vi "Lectura de datos 2.vi"() -> ()   [LabVIEW 2020]
panel:
  out "Graficacion señales":dynamicdata(graph)
  in  "stop":bool
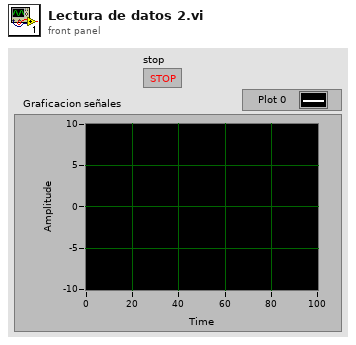
[diagram p1: front panel]
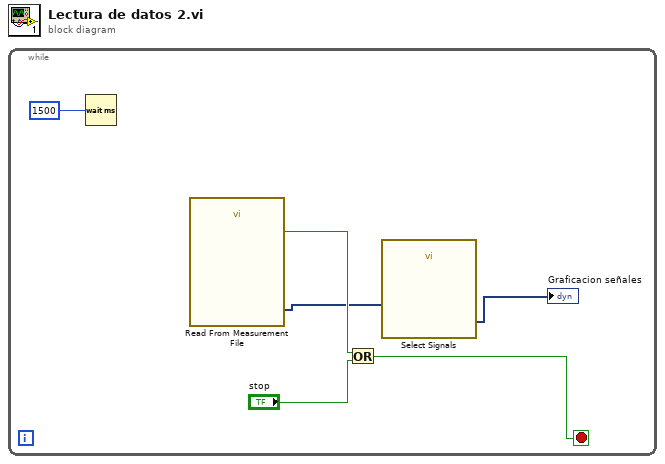
[diagram p0: block diagram]
diagram:
  n1 = while {
    stop <- w3 stop-if-true
    n2 = Wait (ms)(milliseconds to wait=u32 1500 ("millisecond timer value")) -> ()  [unwired: 1 out]
    n3 = call "Read From Measurement File"() -> ("Signals"=w2:dynamicdata, "EOF?"=w5:bool)  [unwired: 6 in, 4 out]
    n4 = Or(x=w5, y="stop") -> (x .or. y?=w3:bool)
    n5 = call "Select Signals"("Signals"=w2) -> ("Signal Out"=→"Graficacion señales":dynamicdata)  [unwired: 9 in, 1 out]
  }
